vi "Thread.Get Priority.vi"(11 "Thread in":refnum<class "Thread.lvclass">) -> (2 "Priority":i32, 3 "Thread out":refnum<class "Thread.lvclass">)   [LabVIEW 2016, in "Thread.lvclass"]
uses:
  Thread.lvclass
  Thread.lvclass/Thread.ctl
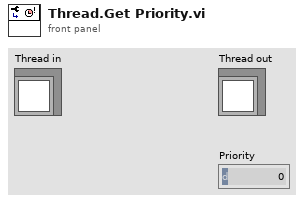
[diagram p1: front panel]
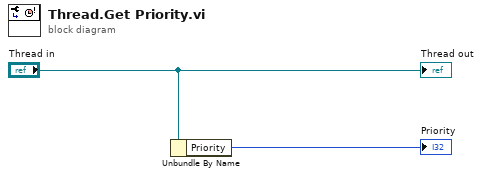
[diagram p0: block diagram]
diagram:
  n1 = Unbundle By Name("Thread in") -> ("Priority"=→"Priority":i32)
  "Thread out" <- "Thread in"
